vi "PID Engine.vi"(7 "State":enum16{"Init", "Get PID"}(ring), 8 "error in (no error)":errorcluster, 11 "PIDs":T2) -> (0 "error out":errorcluster, 2 "String":string, 3 "Cluster":T1 {"Mode" format="%x"; "PID" format="%x"}, 4 "all rows":string[][](array[string]))   [LabVIEW 2011]
uses:
  PID List.ctl
  PID Typedef.ctl
  <vilib>/Utility/file.llb/Read From Spreadsheet File (string).vi
panel:
  out "subarray":string[](array[string])
  out "Table Control":string[][](table)
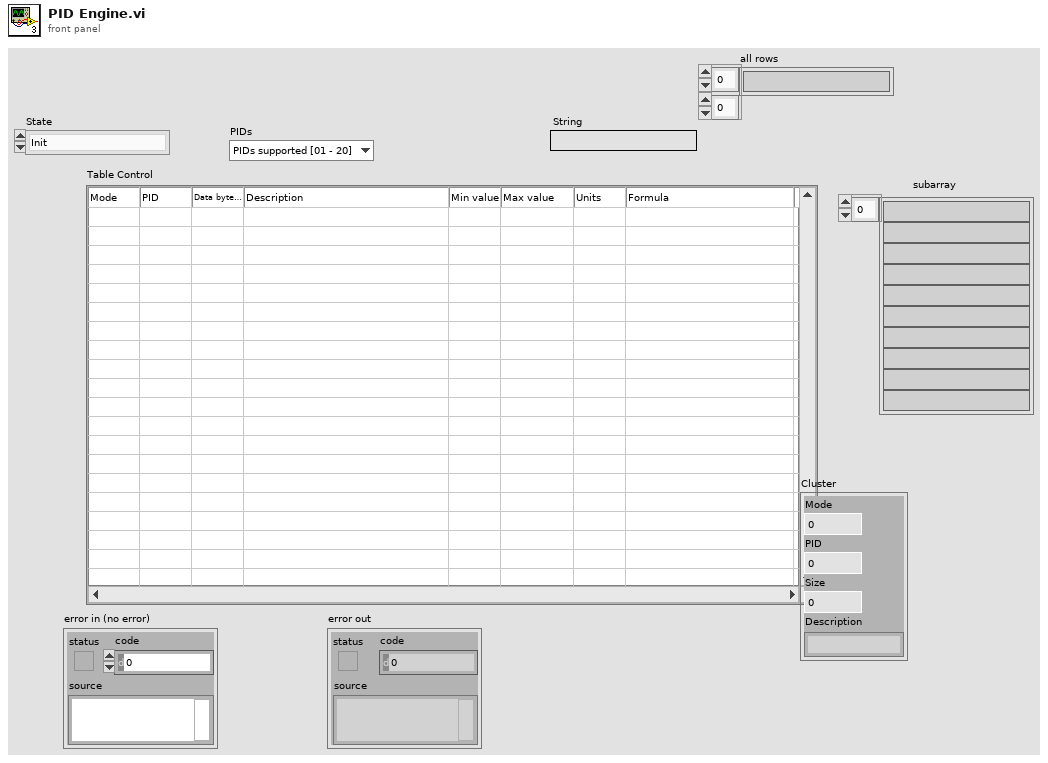
[diagram p1: front panel]
types:
  T1 = typedef "PID Typedef.ctl" = cluster{"Mode":i32, "PID":i32, "Size":i32, "Description":string}
  T2 = typedef "PID List.ctl" = enum16{"PIDs supported [01 - 20]", "Monitor status since DTCs cleared", "Freeze DTC", "Fuel system status", "Caulculated engine load value", "Engine Coolant temperature", "Short term fuel %trim Bank1", "Long term fuel %trim Bank 1", "Short term fuel %trim Bank2", "Long term fuel %trim Bank2", "Fuel pressure", "Intake manifold absolute pressure", "Engine RPM", "Vehicle speed", "timing advance", "Intake air temperature", "MAF air flow rate", "Throttle position", "Commanded secondary air status", "Oxygen sensors present", "bank 1 sensor 1", "Bank 1 sensor 2", "Bank 1 sensor 3", "Bank 1 sensor 4", "Bank 2 sensor 1", "Bank 2 sensor 2", "Bank 2 sensor 3", "Bank 2 sensor 4", "OBD standards this vehicle conforms to", "Oxygen sensor present", "Auxilary input status", "Run time since engine start", "PIDs supported [21-40]", "Distance traveled with malfunction", "Fuel Rail Pressure (manifold)", "Fuel Rail Pressure (gasoline)", "O2S1_WR", "O2S2_WR", "O2S3_WR", "O2S4_WR", "O2S5_WR", "O2S6_WR", "O2S7_WR", "O2S8_WR", "Commanded EGR", "EGR Error", "Commanded evaporative purge", "Fuel Level Input", "# of warm ups since codes cleared", "Distance traveled since codes cleared", "Evap System Vapor Pressure", "Barometric pressure", "O2S1", "O2S2", "O2S3", "O2S4", "O2S5", "O2S6", "O2S7", "O2S8", "Catalyst Temperature B1S1", "Catalyst Temperature B2S1", "Catalyst Temperature B1S2", "Catalyst Temperature B2S2", "PIDs supported [41-60]", "Monitor status this drive cycle", "Control module voltage", "Absolute load value", "Command equivalence ratio", "Relative throttle position", "Ambient air temperature", "Absolute throttle position B", "Absolute throttle position C", "Accelerator pedal position D", "Accelerator pedal position E", "Accelerator pedal position F", "Command throttle actuator", "PIDs supported [61-80]", "Auxilary input / output supported", "Mass air flow sensor", "Engine coolant temperature", "Intake air temperature sensor", "Commanded EGR and EGR Error", "Fuel pressure control system", "Injection pressure control system", "Turbocharger compressor inlet pressure", "Boost pressure control", "Exhaust pressure", "Turbocharger RPM", "Turbocharger temperature", "Turbocharger temperature2", "Vehicle Identification number (VIN)"}
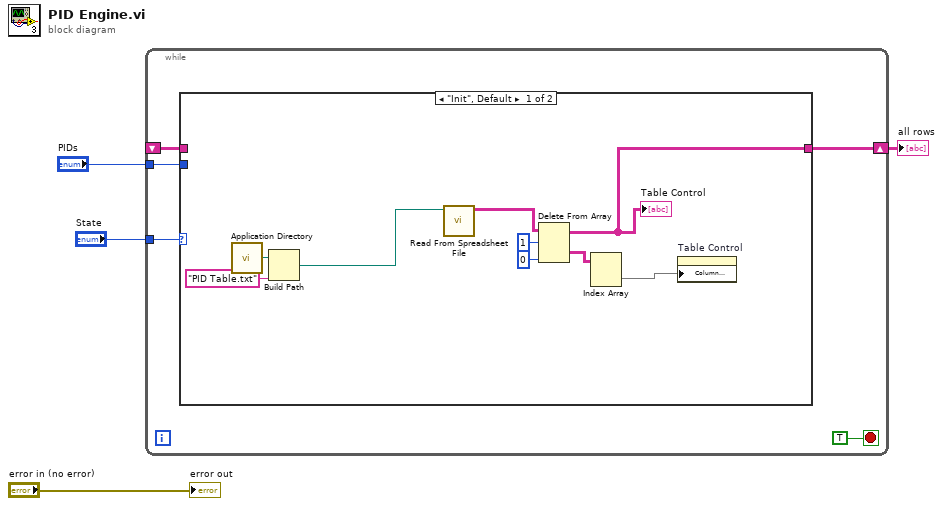
[diagram p0: block diagram]
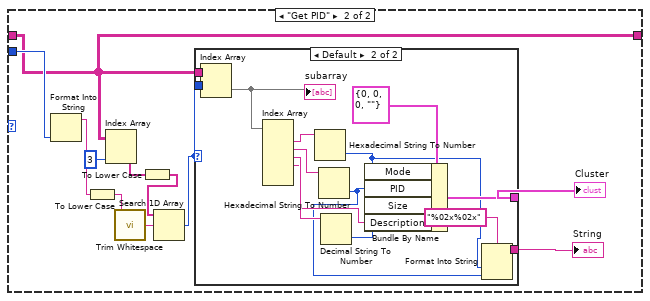
[diagram p2: hidden frame]
diagram:
  n1 = while {
    tunnel: "State" -> [w8]
    tunnel: "PIDs" -> [w7]
    shift-right: [w6] -> w1
    shift-left: _ -> [w5]
    stop <- TRUE stop-if-true
    n2 = case shown="\"Init\", Default" w8 {
      tunnel: w7 -> [_ w27]
      tunnel: [w10 w25] -> w6
      tunnel: w5 -> [_ w25]
      frame "Init", Default {
        n3 = call <vilib>:"Application Directory.vi"() -> ("Application Directory"=w18:path)
        n4 = Build Path(base path=w18, name or relative path="PID Table.txt") -> (appended path=w16:path)
        n5 = call-poly <vilib>:"Read From Spreadsheet File.vi"("file path (dialog if empty)"=w16) -> ("all rows"=w15:string[][])  [unwired: 6 in, 4 out]
        n6 = Delete From Array(array=w15, length=1, index (row)=0) -> (deleted portion=w12:string[][], array with subset deleted=w10:string[][])  [unwired: 1 in]
        "Table Control" <- w10
        n7 = Index Array(array=w12) -> (element=w11:string[])  [unwired: 2 in]
        n8 = property on="Table Control" class="Tbl (strict)"("Column Headers[]"=w11) -> ()  [unwired: 2 in, 2 out]
      }
      frame "Get PID" {
        n9 = Format Into String(w27) -> (resulting string=w26:string)  [unwired: 3 in, 1 out]
        n10 = To Lower Case(string=w26) -> (all lower case string=w21:string)
        n11 = Index Array(array=w25, index (col)=3 ("disabled index (col)")) -> (element=w23:string[])  [unwired: 1 in]
        n12 = call <vilib>:"Trim Whitespace.vi"("string"=w21) -> ("trimmed string"=w19:string)  [unwired: 1 in]
        n13 = To Lower Case(string=w23) -> (all lower case string=w22:string[])
        n14 = Search 1D Array(1D array=w22, element=w19) -> (index of element=w20:i32)  [unwired: 1 in]
        n15 = case shown="Default" w20 {
          tunnel: [_ w41] -> w29
          tunnel: [_ w32] -> w28
          tunnel: w25 -> [_ w31]
          tunnel: w20 -> [_ w30]
          frame -1 {
          }
          frame Default {
            n16 = Index Array(array=w31, index (row)=w30) -> (element=w43:string[])  [unwired: 1 in]
            "subarray" <- w43
            n17 = Index Array(array=w43) -> (element #1=w40:string, element #2=w39:string, element #3=w38:string, element #4=w36:string)  [unwired: 6 in, 2 out]
            n18 = Hexadecimal String To Number(string=w40) -> (number=w34:u32)  [unwired: 2 in, 1 out]
            n19 = Hexadecimal String To Number(string=w39) -> (number=w33:u32)  [unwired: 2 in, 1 out]
            n20 = Decimal String To Number(string=w38) -> (number=w37:i32)  [unwired: 2 in, 1 out]
            n21 = Bundle By Name(cluster=T1 {"Mode"=0, "PID"=0, "Size"=0, "Description"=""} ("Cluster 2"), "Mode"=w34, "PID"=w33, "Size"=w37, "Description"=w36) -> (w41:T1)
            n22 = Format Into String(format string="%02x%02x", w34, w33) -> (resulting string=w32:string)  [unwired: 2 in, 1 out]
          }
        }
        "Cluster" <- w29
        "String" <- w28
      }
    }
  }
  "all rows" <- w1
  "error out" <- "error in (no error)"
